vi "Welch Window.vi"   [LabVIEW 2020, in "NI_AALPro.lvlib"]
doc: "Applies a Welch window to the input signal <B>X</B>. Wire data to the <B>X</B> input to determine the polymorphic instance to use or manually select the instance."
uses:
  NI_AALPro.lvlib
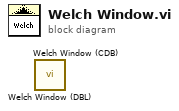
[diagram p0: block diagram]
diagram:
  n1 = call "Welch Window (DBL).vi"() -> ()  [unwired: 10 in, 2 out]
  n2 = call "Welch Window (CDB).vi"() -> ()  [unwired: 10 in, 2 out]
